vi "Change AO Gain (scaled property node) on Fly or Not.vi"() -> ()   [LabVIEW 2015]
doc: "I. Description:\nThis example demonstrates how to output a continuous periodic waveform using an internal sample clock.\n\nII. Instructions for Running:\n1. Select the Physical Channel to correspond to where your signal is output on the DAQ device.\n2. Enter the Minimum and Maximum Voltage Ranges\n3. Specify the Desired Frequency of the output Waveform\n4. Enter the Waveform Information. See the documentation of the Waveform Buffer Generation SubVI for information on each parameter.\n\nIII. Block Diagram Steps:\n1. Create an Analog Output Voltage channel.\n2. Call the DAQmx Timing (Use Waveform) VI which sets the sample clock rate based on the input waveform parameters, and set the sample mode to Continuous.\n3. Write the waveform to the output buffer.\n4. Call the Start VI.\n5. Loop continuously until the user presses the Stop button. Check for errors every 100 ms using the Is Task Done? VI\n6. Clear the Task\n7. Use the popup dialog box to display an error or warning if any.\n\nIV. I/O Connections Overview:\nMake sure your signal output terminal matches the Physical Channel I/O Control. For further connection information, refer to your hardware reference manual."
uses:
  <vilib>/DAQmx/create/channels.llb/DAQmx Create Channel (AO-Voltage-Basic).vi
  <vilib>/Utility/error.llb/DialogType.ctl
  <vilib>/DAQmx/configure/timing.llb/DAQmx Timing (Sample Clock).vi
  <vilib>/DAQmx/write.llb/DAQmx Write (Analog 2D DBL NChan NSamp).vi
  <resource>/objmgr/daqmx.rc
panel:
  in  "AO Gain  Property node":dbl
  in  "physical channels 2":tag="PXI1Slot2/ao0" caption="Output Physical Channels"
  in  "AO Channel":u16(ring)=1536 items=["AO 0"=1536, "AO 1"=1540]
  in  "Gain Setting":u16(ring) items=["0 dB Gain"=0, "20 dB Gain"=2, "40 dB Gain"=4]
  out "Resulting Frequency":dbl format="%.2f"
  in  "Cycles per Buffer":i32=5
  in  "Waveform Type":T1(ring)
  in  "Desired Frequency":dbl=1000.0 format="%.2f"
  in  "Samples per Buffer":dbl=250.0
  in  "Amplitude":dbl=10.0 format="%0.2p"
  out "Waveform Graph":dbl[](graph) caption="Output Waveform"
  in  "Physical Channels":tag="PXI1Slot2/ao0:1"
  in  "Minimum Value":dbl=-10.0 format="%0.2f"
  in  "Maximum Value":dbl=10.0 format="%0.2f"
  in  "stop":bool
  # "For instructions, select Help>>Show Context Help"
  # "Channel Parameters"
  # "Timing Parameters"
  # "Waveform Information"
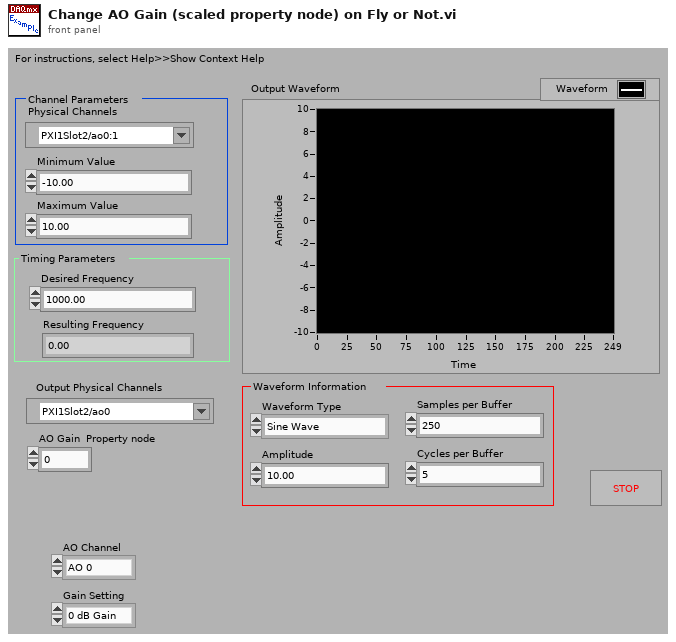
[diagram p1: front panel]
types:
  T1 = enum16{"Sine Wave", "Triangle Wave", "Square Wave", "Sawtooth Wave"}
  T2 = typedef "DialogType.ctl" = u16
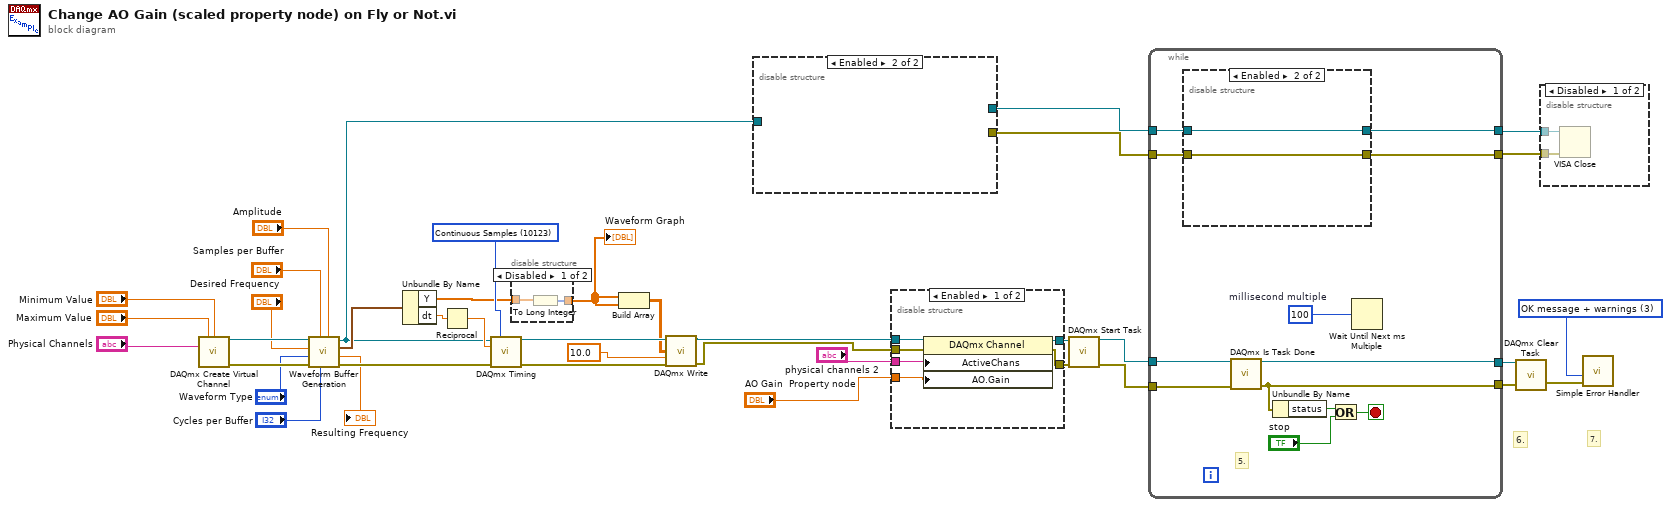
[diagram p0: block diagram]
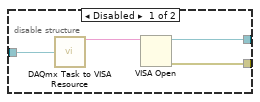
[diagram p3: hidden frame]
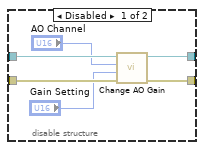
[diagram p6: hidden frame]
diagram:
  w12 = 10123 items=["Finite Samples"=10178, "Continuous Samples"=10123, "Hardware Timed Single Point"=12522] ("sample mode")
  w30 = T2 3 items=["no dialog", "OK message", "continue or stop message", "OK message + warnings", "continue/stop + warnings"] ("type of dialog (OK msg:1)")
  # "7."
  # "6."
  n1 = call-poly <vilib>:"DAQmx Create Virtual Channel.vi"("maximum value"="Maximum Value", "minimum value"="Minimum Value", "physical channels"="Physical Channels") -> ("task out"=w26:refnum<k21>, "error out"=w25:errorcluster)  [unwired: 11 in]
  n2 = call "Waveform Buffer Generation.vi"("Amplitude"="Amplitude", "Cycles per Buffer"="Cycles per Buffer", "Samples per Buffer"="Samples per Buffer", "error in (no error)"=w25, "Waveform Type"="Waveform Type", "Desired Frequency"="Desired Frequency", "task/channels in"=w26) -> ("error out"=w27:errorcluster, "Resulting Frequency"=→"Resulting Frequency":dbl, "Waveform"=w15:waveform(dbl), "task out"=w9:refnum<k21>)  [unwired: 1 out]
  n3 = Unbundle By Name(w15) -> ("Y"=w1:dbl[], "dt"=w14:dbl)
  n4 = Reciprocal(x=w14) -> (1/x=w13:dbl)
  n5 = call-poly <vilib>:"DAQmx Timing.vi"("task/channels in"=w9, "sample mode"=w12, "rate"=w13, "error in"=w27) -> ("task out"=w33:refnum<k21>, "error out"=w32:errorcluster)  [unwired: 10 in]
  n6 = disable-structure shown="Disabled" {
    disable-tunnel: [w41 w42] -> w2
    disable-tunnel: w1 -> [w40 w42]
    frame Disabled {
      n7 = To Long Integer(number=w40) -> (32bit integer=w41:i32[])
    }
    frame Enabled {
    }
  }
  "Waveform Graph" <- w2
  n8 = Build Array(w2, w2) -> (w11:dbl[][])
  n9 = call-poly <vilib>:"DAQmx Write.vi"("task/channels in"=w33, "data"=w11, "timeout"=10.0 ("Wirite Timeout"), "error in"=w32) -> ("task out"=w7:refnum<k21>, "error out"=w4:errorcluster)  [unwired: 9 in, 1 out]
  n10 = disable-structure shown="Enabled" {
    disable-tunnel: [w46 _] -> w19
    disable-tunnel: [w45 _] -> w18
    disable-tunnel: w9 -> [w44 _]
    frame Disabled {
      n11 = call "DAQmx Task to VISA Resource.vi"("task out"=w44) -> ("VISAName"=w43:string)
      n12 = VISA Open(VISA resource name=w43) -> (VISA resource name=w46:refnum<visa-resource-name>, error out=w45:errorcluster)  [unwired: 4 in]
    }
    frame Enabled {
    }
  }
  n13 = disable-structure shown="Enabled" {
    disable-tunnel: "AO Gain  Property node" -> [w52 _]
    disable-tunnel: "physical channels 2" -> [w51 _]
    disable-tunnel: w7 -> [w50 w54]
    disable-tunnel: [w49 w54] -> w6
    disable-tunnel: [w48 w53] -> w5
    disable-tunnel: w4 -> [w47 w53]
    frame Enabled {
      n14 = property class="DAQmx Channel"(reference=w50, error in=w47, "ActiveChans"=w51, "AO.Gain"=w52) -> (reference out=w49:refnum<k21>, error out=w48:errorcluster)
    }
    frame Disabled {
    }
  }
  n15 = call <vilib>:"DAQmx Start Task.vi"("task/channels in"=w6, "error in"=w5) -> ("task out"=w31:refnum<k21>, "error out"=w35:errorcluster)  [unwired: 12 in]
  n16 = while {
    tunnel: w31 -> [w66]
    tunnel: [w65] -> w29
    tunnel: w35 -> [w64]
    tunnel: [w63] -> w28
    tunnel: w19 -> [w58]
    tunnel: w18 -> [w57]
    tunnel: [w56] -> w17
    tunnel: [w55] -> w16
    stop <- w61 stop-if-true
    w62 = u32 100  # millisecond multiple
    # "5."
    n17 = disable-structure shown="Enabled" {
      disable-tunnel: w58 -> [w72 w74]
      disable-tunnel: w57 -> [w71 w73]
      disable-tunnel: [w70 w74] -> w56
      disable-tunnel: [w69 w73] -> w55
      frame Disabled {
        n18 = call "Change AO Gain.vi"("error in"=w71, "Gain Setting"="Gain Setting", "AO Channel"="AO Channel", "VISA resource name 2"=w72) -> ("error out"=w69:errorcluster, "VISA resource name"=w70:refnum<visa-resource-name>)  [unwired: 4 in]
      }
      frame Enabled {
      }
    }
    n19 = call <vilib>:"DAQmx Is Task Done.vi"("task/channels in"=w66, "error in"=w64) -> ("task out"=w65:refnum<k21>, "error out"=w63:errorcluster)  [unwired: 11 in, 1 out]
    n20 = Unbundle By Name(w63) -> ("status"=w60:bool)
    n21 = Or(x=w60, y="stop") -> (x .or. y?=w61:bool)
    n22 = Wait Until Next ms Multiple(millisecond multiple=w62) -> ()  [unwired: 1 out]
  }
  n23 = call <vilib>:"DAQmx Clear Task.vi"("task in"=w29, "error in"=w28) -> ("error out"=w39:errorcluster)  [unwired: 13 in]
  n24 = disable-structure shown="Disabled" {
    disable-tunnel: w17 -> [w76 _]
    disable-tunnel: w16 -> [w75 _]
    frame Disabled {
      n25 = VISA Close(VISA resource name=w76, error in (no error)=w75) -> ()  [unwired: 1 out]
    }
    frame Enabled {
    }
  }
  n26 = call <vilib>:"Simple Error Handler.vi"("type of dialog (OK msg:1)"=w30, "error in (no error)"=w39) -> ()  [unwired: 3 in, 5 out]
